vi "dR_R.vi"(9 "Image Type":T1 items=["Grayscale (U8)", "Grayscale (I16)", "Grayscale (SGL)", "Complex (CSG)", "RGB (U32)", "HSL (U32)", "RGB (U64)", "Grayscale (U16)"], 10 "initial frame NO.":i32=10, 11 "imaging input":T2[](array[typedef])) -> (3 "imaging output":T2[](array[typedef]))   [LabVIEW 2011]
uses:
  <vilib>/vision/Image Controls.llb/IMAQ Image.ctl
  <vilib>/vision/NI_Vision_Development_Module.lvlib
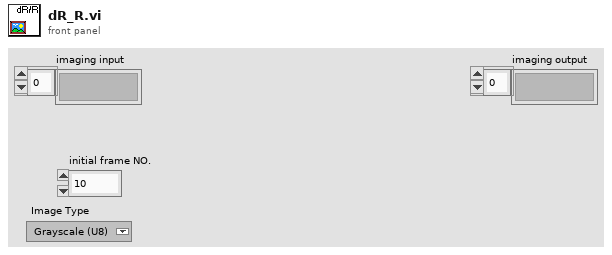
[diagram p1: front panel]
types:
  T1 = typedef "Image Type" = u32
  T2 = typedef "IMAQ Image.ctl" = refnum<image>
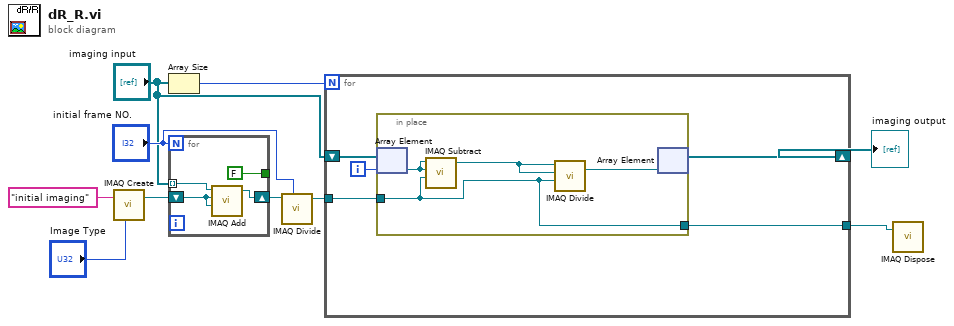
[diagram p0: block diagram]
diagram:
  n1 = call "IMAQ Create"("Image Name"="initial imaging", "Image Type"="Image Type") -> ("New Image"=w7:T2)  [unwired: 3 in, 1 out]
  n2 = Array Size(array="imaging input") -> (size(s)=w5:i32)
  n3 = for {
    N: "initial frame NO." -> [_]
    tunnel: "imaging input" -> [w14] mode=indexing
    shift-right: [w13] -> w9
    shift-left: w7 -> [w12]
    tunnel: [FALSE ("标志")] -> _
    n4 = call "IMAQ Add"("Image Src A"=w14, "Image Dst"=w12, "Image Src B"=w12) -> ("Image Dst Out"=w13:T2)  [unwired: 4 in, 1 out]
  }
  n5 = call "IMAQ Divide"("Image Src A"=w9, "Constant"="initial frame NO.") -> ("Image Dst Out"=w4:T2)  [unwired: 5 in, 1 out]
  n6 = for {
    N: w5 -> [_]
    tunnel: w4 -> [w17]
    shift-right: [w16] -> w3
    shift-left: "imaging input" -> [w19]
    tunnel: [w15] -> w1
    i -> [w18]
    n7 = in-place {
      in-place-border: w17 -> [w20]
      in-place-border: [w20] -> w15
      n8 = in-place-array #1(w19, w18) -> (w22:T2)
      n9 = call "IMAQ Subtract"("Image Src A"=w22, "Image Dst"=w22, "Image Src B"=w20) -> ("Image Dst Out"=w21:T2)  [unwired: 4 in, 1 out]
      n10 = call "IMAQ Divide"("Image Src A"=w21, "Image Dst"=w21, "Image Src B"=w20) -> ("Image Dst Out"=w23:T2)  [unwired: 4 in, 1 out]
      n11 = in-place-array #1(w23) -> (w16:T2[])  [unwired: 1 out]
    }
  }
  "imaging output" <- w3
  n12 = call "IMAQ Dispose"("Image"=w1) -> ()  [unwired: 5 in, 1 out]
